vi "Show User Interface.vi"(8 "error in (no error)":errorcluster, 9 "Process VI Refnums":refnum<vi>[](array[refnum]), 10 "Show UI":bool, 11 "My.SMO.UI":refnum<class "My.SMO.UI.lvclass">) -> (0 "error out":errorcluster, 3 "My.SMO.UI out":refnum<class "My.SMO.UI.lvclass">)   [LabVIEW 2016, in "My.SMO.UI.lvclass"]
doc: "JKI State Machine Objects (SMO) 1.0.0.5\nJKI - JKI\nCopyright (c) 2016, JKI"
uses:
  My.SMO.UI.lvclass
  <vilib>/JKI/JKI SMO/SMO.UI/SMO.UI.lvclass
  <vilib>/JKI/JKI SMO/SMO/SMO.lvclass
  C:/Program Files (x86)/National Instruments/LabVIEW 2016/vi.lib/JKI/JKI SMO/SMO/SMO.lvclass
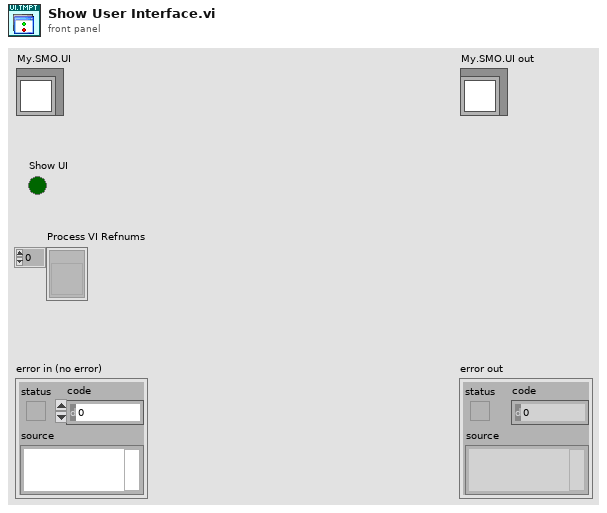
[diagram p1: front panel]
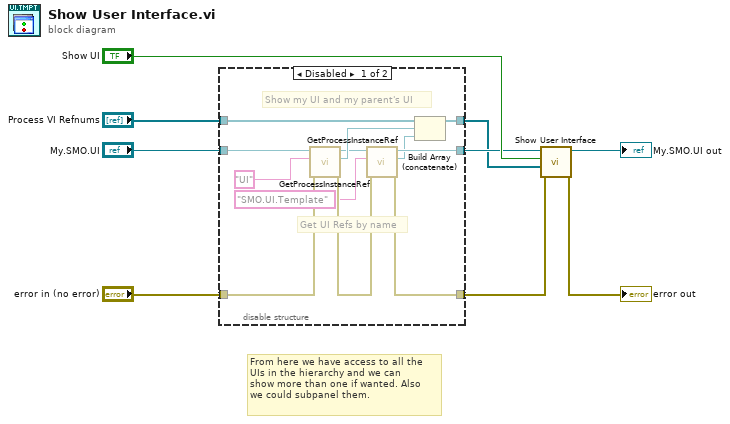
[diagram p0: block diagram]
diagram:
  # "From here we have access to all the\nUIs in the hierarchy and we can \nshow more than one if wanted. Also\nwe could subpanel them."
  n1 = disable-structure shown="Disabled" {
    disable-tunnel: "My.SMO.UI" -> [w21 w24]
    disable-tunnel: [w14 w24] -> w5
    disable-tunnel: "error in (no error)" -> [w20 w23]
    disable-tunnel: [w12 w23] -> w3
    disable-tunnel: "Process VI Refnums" -> [w18 w22]
    disable-tunnel: [w16 w22] -> w1
    frame Disabled {
      # "Get UI Refs by name"
      # "Show my UI and my parent's UI"
      n2 = call <vilib>:"GetProcessInstanceRef.vi"("error in (no error)"=w20, "Process Name"="UI", "SMO"=w21) -> ("error out"=w13:errorcluster, "Process VI Refnum"=w17:refnum<vi>, "SMO out"=w15:refnum<class "My.SMO.UI.lvclass">)  [unwired: 6 in]
      n3 = call <vilib>:"GetProcessInstanceRef.vi"("error in (no error)"=w13, "Process Name"="SMO.UI.Template", "SMO"=w15) -> ("error out"=w12:errorcluster, "Process VI Refnum"=w10:refnum<vi>, "SMO out"=w14:refnum<class "My.SMO.UI.lvclass">)  [unwired: 6 in]
      n4 = Build Array (concatenate)(w18, w17, w10) -> (w16:refnum<vi>[])
    }
    frame Enabled {
      # "Show only my UI"
    }
  }
  n5 = call-parent "Show User Interface.vi"("error in (no error)"=w3, "Process VI Refnums"=w1, "Show UI"="Show UI", "SMO.UI"=w5) -> ("error out"=→"error out":errorcluster, "SMO.UI out"=→"My.SMO.UI out":refnum<class "My.SMO.UI.lvclass">)  [unwired: 6 in]
